vi "Lookup String.vi"(8 "error in (no error)":errorcluster, 11 "Locale String":T1) -> (0 "error out":errorcluster, 3 "String":string)   [LabVIEW 2018, in "Scripting.lvlib"]
uses:
  Scripting.lvlib
  Locale-Strings.ctl
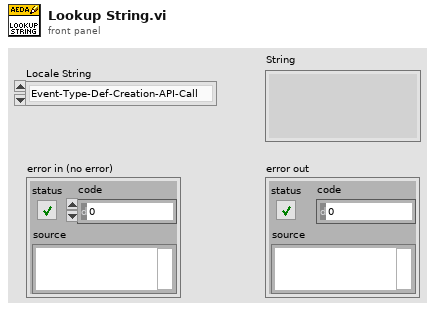
[diagram p1: front panel]
types:
  T1 = typedef "Scripting.lvlib/Locale-Strings.ctl" = enum16{"Event-Type-Def-Creation-API-Call"}
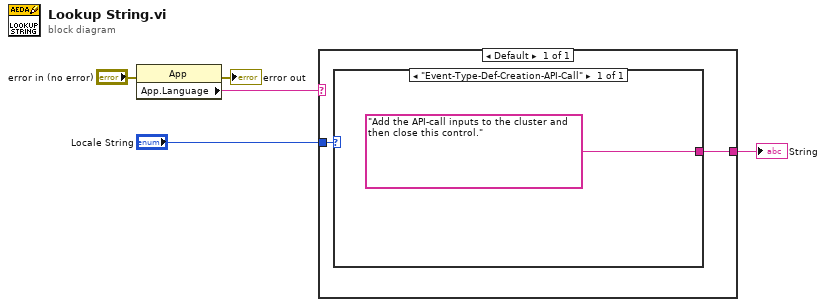
[diagram p0: block diagram]
diagram:
  n1 = property class="App"(error in="error in (no error)") -> (error out=→"error out":errorcluster, "App.Language"=w2:string)  [unwired: 1 in, 1 out]
  n2 = case shown="Default" w2 {
    tunnel: "Locale String" -> [w7]
    tunnel: [w6] -> w1
    frame Default {
      n3 = case shown="\"Event-Type-Def-Creation-API-Call\"" w7 {
        tunnel: ["Add the API-call inputs to the cluster and then close this control."] -> w6
        frame "Event-Type-Def-Creation-API-Call" {
        }
      }
    }
  }
  "String" <- w1
